vi "ACQ device create counters.vi"(7 "Config Counter channels":T1, 10 "device in":tag) -> (0 "DAQ en X":tag, 1 "DAQ en Y":tag, 2 "DAQ gen":tag, 3 "DAQ gen out":tag)   [LabVIEW 2013]
uses:
  Kontrolki/KartaDAQ/ACQ counter channel config.ctl
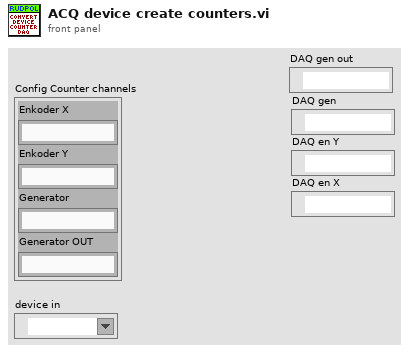
[diagram p1: front panel]
types:
  T1 = typedef "ACQ counter channel config.ctl" = cluster{"Enkoder X":string, "Enkoder Y":string, "Generator":string, "Generator OUT":string}
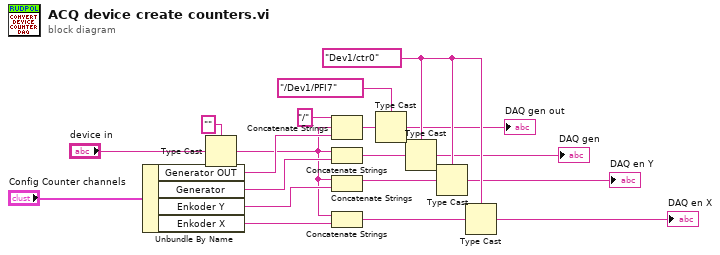
[diagram p0: block diagram]
diagram:
  w7 = tag "Dev1/ctr0" ("counter X")
  n1 = Unbundle By Name("Config Counter channels") -> ("Generator OUT"=w16:string, "Generator"=w17:string, "Enkoder Y"=w18:string, "Enkoder X"=w19:string)
  n2 = Type Cast(type="", x="device in") -> (*(type *) &x=w14:string)
  n3 = Concatenate Strings("/", w14, w16) -> (w11:string)
  n4 = Concatenate Strings(w14, w17) -> (w10:string)
  n5 = Concatenate Strings(w14, w18) -> (w9:string)
  n6 = Concatenate Strings(w14, w19) -> (w8:string)
  n7 = Type Cast(type=tag "/Dev1/PFI7" ("CO.Pulse.Term"), x=w11) -> (*(type *) &x=→"DAQ gen out":tag)
  n8 = Type Cast(type=w7, x=w10) -> (*(type *) &x=→"DAQ gen":tag)
  n9 = Type Cast(type=w7, x=w9) -> (*(type *) &x=→"DAQ en Y":tag)
  n10 = Type Cast(type=w7, x=w8) -> (*(type *) &x=→"DAQ en X":tag)
